vi "Execute 7z bat.vi"(8 "error in (no error)":errorcluster, 11 "PostBuildSupport in":refnum<class "PostBuildSupport.lvclass">) -> (0 "error out":errorcluster, 3 "PostBuildSupport out":refnum<class "PostBuildSupport.lvclass">)   [LabVIEW 2016, in "PostBuildSupport.lvclass"]
uses:
  PostBuildSupport.lvclass
  PostBuildSupport.lvclass/PostBuildSupport.ctl
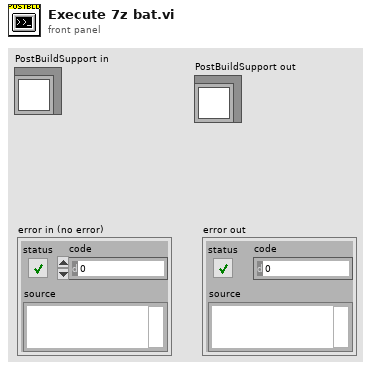
[diagram p1: front panel]
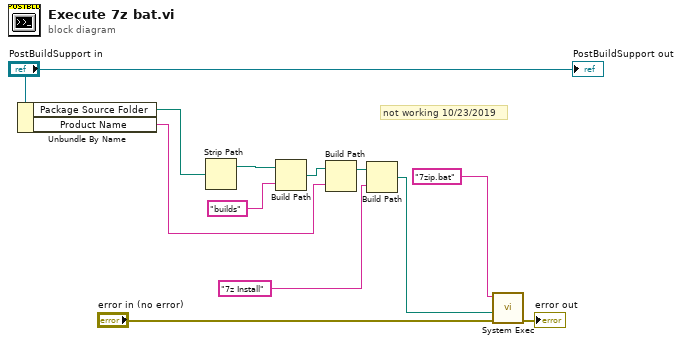
[diagram p0: block diagram]
diagram:
  # "not working 10/23/2019"
  n1 = Unbundle By Name("PostBuildSupport in") -> ("Package Source Folder"=w7:path, "Product Name"=w1:string)
  n2 = Strip Path(path=w7) -> (stripped path=w11:path)  [unwired: 1 out]
  n3 = Build Path(base path=w11, name or relative path="builds") -> (appended path=w2:path)
  n4 = Build Path(base path=w2, name or relative path=w1) -> (appended path=w5:path)
  n5 = Build Path(base path=w5, name or relative path="7z Install") -> (appended path=w4:path)
  n6 = call <vilib>:"System Exec.vi"("error in (no error)"="error in (no error)", "working directory"=w4, "command line"="7zip.bat" ("name or relative path")) -> ("error out"=→"error out":errorcluster)  [unwired: 5 in, 3 out]
  "PostBuildSupport out" <- "PostBuildSupport in"
